vi "PRTtagFGV.vi"(10 "Action":T1(ring), 11 "PRT in":string) -> (3 "PRT out":string)   [LabVIEW 2012, in "StimulCtrls.lvlib"]
uses:
  StimulCtrls.lvlib
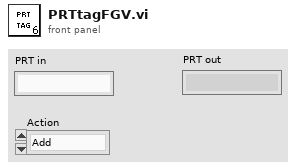
[diagram p1: front panel]
types:
  T1 = enum16{"Add", "Set", "Del", "Update", "Get", "Initial", "GetSize"}
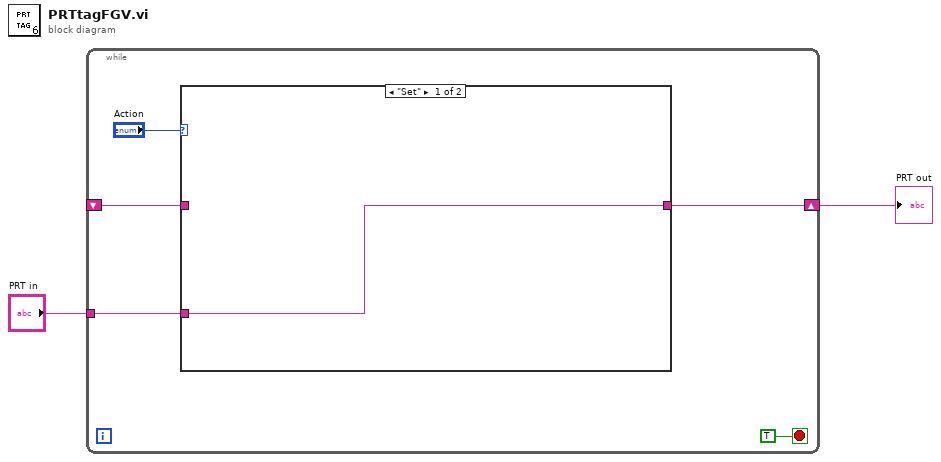
[diagram p0: block diagram]
diagram:
  n1 = while {
    shift-right: [w4] -> w1
    shift-left: _ -> [w5]
    tunnel: "PRT in" -> [w3]
    stop <- TRUE stop-if-true
    n2 = case shown="\"Set\"" "Action" {
      tunnel: w5 -> [_ w9]
      tunnel: [w8 w9] -> w4
      tunnel: w3 -> [w8 _]
      frame "Set" {
      }
      frame "Get", Default {
      }
    }
  }
  "PRT out" <- w1
